vi "LVIS_Result.vi"(5 "LastEventMeas?":bool, 7 "LastTestMeas?":bool, 8 "Error In":errorcluster, 9 "Log Step?":bool, 10 "Status":string, 11 "Value":string) -> (0 "Error Out":errorcluster, 2 "Result":T1, 3 "IS_Data":string[](array[string]))   [LabVIEW 2015]
doc: "If applicable, derives the measurement status. If LastTestMeas, derives the test status. If LastEventMeas, derives the event status."
uses:
  Globals/LVIS_IsGlobal.vi
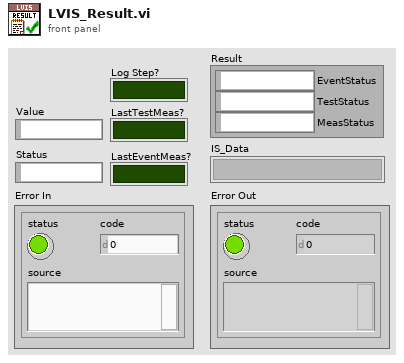
[diagram p1: front panel]
types:
  T1 = cluster{"EventStatus":string, "TestStatus":string, "MeasStatus":string}
  T2 = cluster{"MeasName":string, "MeasDateTime":string, "MeasStatus":string, "MeasClientID":string, "IS_MeasID":string, "MeasType":string, "MeasValue":string, "LL":string, "LL Comp":string, "HL":string, "HL Comp":string, "Units":string, "MeasMeta":string}
  T3 = cluster{"TestName":string, "TestDateTime":string, "TestStatus":string, "TestClientID":string, "IS_TestID":string, "TestMeta":string}
  T4 = cluster{"EventName":string, "EventStart":string, "EventStop":string, "EventStatus":string, "EventClientID":string, "IS_EventID":string, "EventMeta":string, "ProductLine":string, "ProcessName":string, "Station":string, "Operator":string, "SN":string, "Model":string, "Manufacturer":string}
  T5 = cluster{"EventInfo":cluster{"EventName":string, "EventStart":string, "EventStop":string, "EventStatus":string, "EventClientID":string, "IS_EventID":string, "EventMeta":string, "ProductLine":string, "ProcessName":string, "Station":string, "Operator":string, "SN":string, "Model":string, "Manufacturer":string}, "TestInfo":cluster{"TestName":string, "TestDateTime":string, "TestStatus":string, "TestClientID":string, "IS_TestID":string, "TestMeta":string}, "MeasInfo":cluster{"MeasName":string, "MeasDateTime":string, "MeasStatus":string, "MeasClientID":string, "IS_MeasID":string, "MeasType":string, "MeasValue":string, "LL":string, "LL Comp":string, "HL":string, "HL Comp":string, "Units":string, "MeasMeta":string}}
  T6 = cluster{"EventInfo":cluster{"EventName":string, "EventStart":string, "EventStop":string, "EventStatus":string, "EventClientID":string, "IS_EventID":string, "EventMeta":string, "ProductLine":string, "ProcessName":string, "Station":string, "Operator":string, "SN":string, "Model":string, "Manufacturer":string}, "TestInfo":cluster{"TestName":string, "TestDateTime":string, "TestStatus":string, "TestClientID":string, "IS_TestID":string, "TestMeta":string}, "MeasInfo":cluster{"MeasName":string, "MeasDateTime":string, "MeasStatus":string, "MeasClientID":string, "IS_MeasID":string, "MeasMeta":string, "MeasType":string, "MeasValue":string, "LL":string, "LL Comp":string, "HL":string, "HL Comp":string, "Units":string}}[]
  T7 = cluster{"EventInfo":cluster{"EventName":string, "EventStart":string, "EventStop":string, "EventStatus":string, "EventClientID":string, "IS_EventID":string, "EventMeta":string, "ProductLine":string, "ProcessName":string, "Station":string, "Operator":string, "SN":string, "Model":string, "Manufacturer":string}, "TestInfo":cluster{"TestName":string, "TestDateTime":string, "TestStatus":string, "TestClientID":string, "IS_TestID":string, "TestMeta":string}, "MeasInfo":cluster{"MeasName":string, "MeasDateTime":string, "MeasStatus":string, "MeasClientID":string, "IS_MeasID":string, "MeasType":string, "MeasValue":string, "LL":string, "LL Comp":string, "HL":string, "HL Comp":string, "Units":string, "MeasMeta":string}}[]
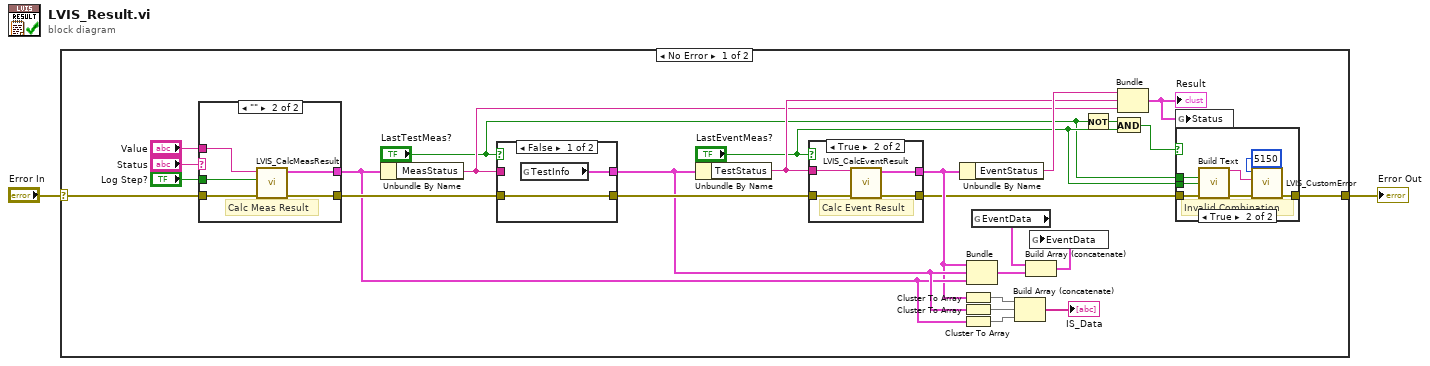
[diagram p0: block diagram]
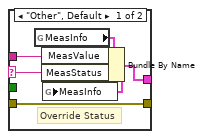
[diagram p3: hidden frame]
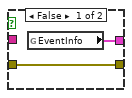
[diagram p4: hidden frame]
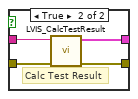
[diagram p5: hidden frame]
diagram:
  n1 = case shown="No Error" "Error In" {
    selector: "Error In" -> [w23 w59]
    tunnel: [w9 w59] -> w1
    frame No Error {
      n2 = case shown="\"\"" "Status" {
        selector: "Status" -> [w37 _]
        tunnel: [w40 w46] -> w26
        tunnel: "Value" -> [w38 w45]
        tunnel: [w39 w44] -> w19
        tunnel: w23 -> [w40 w43]
        tunnel: "Log Step?" -> [_ w42]
        frame "Other", Default {
          # "Override Status"
          n3 = global read "LVIS_IsGlobal.vi" "MeasInfo"() -> (w41:T2)
          n4 = Bundle By Name(cluster=w41, "MeasValue"=w38, "MeasStatus"=w37) -> (w39:T2)
          n5 = global write "LVIS_IsGlobal.vi" "MeasInfo"(w39) -> ()
        }
        frame "" {
          # "Calc Meas Result"
          n6 = call "LVIS_CalcMeasResult.vi"("Error In"=w43, "Log Step?"=w42, "Value"=w45) -> ("Error out"=w46:errorcluster, "MeasInfo"=w44:T2)  [unwired: 7 in]
        }
      }
      n7 = Unbundle By Name(w19) -> ("MeasStatus"=w11:string)
      n8 = case shown="False" "LastTestMeas?" {
        tunnel: w26 -> [w54 w58]
        tunnel: [w54 w57] -> w24
        tunnel: [w53 w56] -> w20
        tunnel: w11 -> [_ w55]
        frame False {
          n9 = global read "LVIS_IsGlobal.vi" "TestInfo"() -> (w53:T3)
        }
        frame True {
          # "Calc Test Result"
          n10 = call "LVIS_CalcTestResult.vi"("Error In"=w58, "MeasStatus"=w55) -> ("Error out"=w57:errorcluster, "TestInfo"=w56:T3)  [unwired: 8 in]
        }
      }
      n11 = Unbundle By Name(w20) -> ("TestStatus"=w12:string)
      n12 = case shown="True" "LastEventMeas?" {
        tunnel: w24 -> [w47 w52]
        tunnel: [w47 w51] -> w10
        tunnel: [w48 w50] -> w14
        tunnel: w12 -> [_ w49]
        frame False {
          n13 = global read "LVIS_IsGlobal.vi" "EventInfo"() -> (w48:T4)
        }
        frame True {
          # "Calc Event Result"
          n14 = call "LVIS_CalcEventResult.vi"("Error In"=w52, "TestStatus"=w49) -> ("Error out"=w51:errorcluster, "EventInfo"=w50:T4)  [unwired: 8 in]
        }
      }
      n15 = Unbundle By Name(w14) -> ("EventStatus"=w13:string)
      n16 = Cluster To Array(cluster=w14) -> (array=w18:string[])
      n17 = Cluster To Array(cluster=w20) -> (array=w17:string[])
      n18 = Cluster To Array(cluster=w19) -> (array=w16:string[])
      n19 = Bundle("EventInfo"=w14, "TestInfo"=w20, "MeasInfo"=w19) -> (w21:T5)  [unwired: 1 in]
      n20 = global read "LVIS_IsGlobal.vi" "EventData"() -> (w28:T6)
      n21 = Build Array (concatenate)(w18, w17, w16) -> (→"IS_Data":string[])
      n22 = Build Array (concatenate)(w28, w21) -> (w27:T7)
      n23 = global write "LVIS_IsGlobal.vi" "EventData"(w27) -> ()
      n24 = Not(x="LastTestMeas?") -> (.not. x?=w6:bool)
      n25 = And(x=w6, y="LastEventMeas?") -> (x .and. y?=w8:bool)
      n26 = Bundle("EventStatus"=w13, "TestStatus"=w12, "MeasStatus"=w11) -> (w3:T1)  [unwired: 1 in]
      "Result" <- w3
      n27 = global write "LVIS_IsGlobal.vi" "Status"(w3) -> ()
      n28 = case shown="True" w8 {
        tunnel: w10 -> [w29 w34]
        tunnel: [w29 w35] -> w9
        tunnel: "LastEventMeas?" -> [_ w31]
        tunnel: "LastTestMeas?" -> [_ w30]
        frame False {
        }
        frame True {
          # "Invalid Combination"
          n29 = call "Build Text"("LTM"=w30, "LEM"=w31, "error in (no error)"=w34) -> ("Result"=w32:string, "error out"=w33:errorcluster)  [unwired: 11 in]
          n30 = call "LVIS_CustomError.vi"("error in (no error)"=w33, "Addiitional Info"=w32, "Code"=5150) -> ("error out"=w35:errorcluster)  [unwired: 8 in]
        }
      }
    }
    frame Error {
    }
  }
  "Error Out" <- w1
